vi "Random Generator.vi"(11 "Max. Value":dbl) -> (3 "Random Value":dbl)   [LabVIEW 2014]
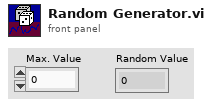
[diagram p1: front panel]
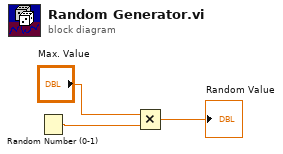
[diagram p0: block diagram]
diagram:
  n1 = Random Number (0-1)() -> (number: 0 to 1=w2:dbl)
  n2 = Multiply(x="Max. Value", y=w2) -> (x*y=→"Random Value":dbl)
